vi "Required LV Version.vi"(8 "error in (no error)":errorcluster, 11 "Build Package Item in":refnum<class "Build Package Item.lvclass">) -> (0 "error out":errorcluster, 1 "64 Bit?":bool, 2 "LV Year":u32)   [LabVIEW 2019, in "VIPM.lvlib" / "Build Package Item.lvclass"]
uses:
  Build Package Item.lvclass
  <vilib>/xml/NI_XML.lvlib
  <vilib>/xml/Close Reference(Node).vi
  <vilib>/xml/Load XML File.vi
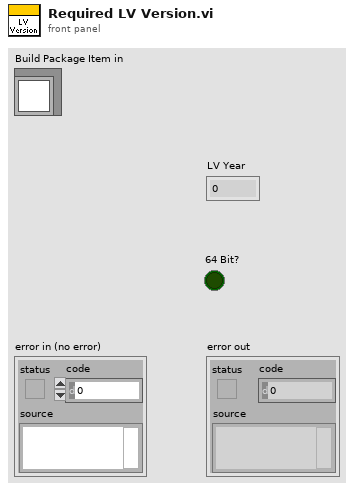
[diagram p1: front panel]
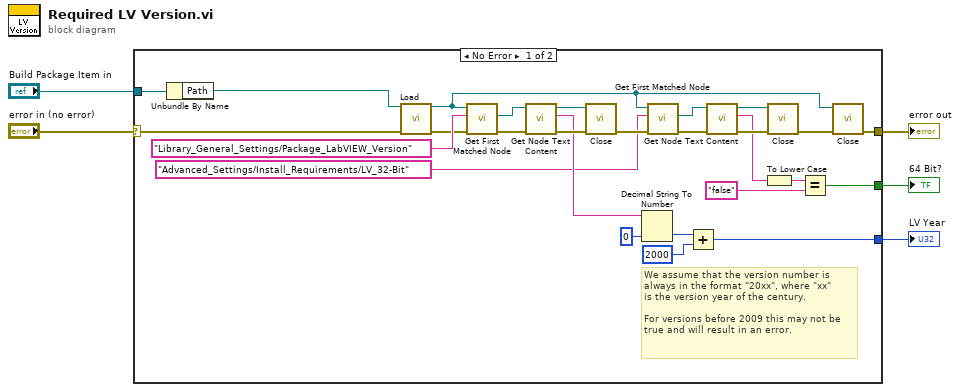
[diagram p0: block diagram]
diagram:
  n1 = case shown="No Error" "error in (no error)" {
    selector: "error in (no error)" -> [w25 w33]
    tunnel: [w24 w33] -> w4
    tunnel: [w20 _] -> w3
    tunnel: "Build Package Item in" -> [w19 _]
    tunnel: [w6 _] -> w1
    frame No Error {
      # "We assume that the version number is\nalways in the format \"20xx\", where \"xx\"\nis the version year of the century.\n\nFor versions before 2009 this may not be\ntrue and will result in an error."
      n2 = Unbundle By Name(w19) -> ("Path"=w18:path)
      n3 = call-poly <vilib>:"Load.vi"("path to XML document"=w18, "error in (no error)"=w25) -> ("DOM document out"=w10:refnum<k20>, "error out"=w31:errorcluster)  [unwired: 11 in, 1 out]
      n4 = call <vilib>:"Get First Matched Node.vi"("error in (no error)"=w31, "XPath expression"="Library_General_Settings/Package_LabVIEW_Version", "node in"=w10) -> ("error out"=w29:errorcluster, "node result"=w30:refnum<k20>)  [unwired: 6 in, 1 out]
      n5 = call <vilib>:"Get Node Text Content.vi"("error in (no error)"=w29, "node in"=w30) -> ("error out"=w28:errorcluster, "node text"=w26:string, "node out"=w27:refnum<k20>)  [unwired: 7 in]
      n6 = call-poly <vilib>:"Close.vi"("error in (no error)"=w28, "node"=w27) -> ("error out"=w16:errorcluster)  [unwired: 7 in]
      n7 = Decimal String To Number(string=w26, default (0L)=u32 0 ("default (0 I32)")) -> (number=w22:u32)  [unwired: 1 in, 1 out]
      n8 = call <vilib>:"Get First Matched Node.vi"("error in (no error)"=w16, "XPath expression"="Advanced_Settings/Install_Requirements/LV_32-Bit", "node in"=w10) -> ("error out"=w17:errorcluster, "node result"=w11:refnum<k20>)  [unwired: 6 in, 1 out]
      n9 = Add(x=w22, y=u32 2000) -> (x+y=w20:u32)
      n10 = call <vilib>:"Get Node Text Content.vi"("error in (no error)"=w17, "node in"=w11) -> ("error out"=w15:errorcluster, "node text"=w9:string, "node out"=w14:refnum<k20>)  [unwired: 7 in]
      n11 = To Lower Case(string=w9) -> (all lower case string=w8:string)
      n12 = call-poly <vilib>:"Close.vi"("error in (no error)"=w15, "node"=w14) -> ("error out"=w13:errorcluster)  [unwired: 7 in]
      n13 = Equal?(x=w8, y="false") -> (x = y?=w6:bool)
      n14 = call-poly <vilib>:"Close.vi"("error in (no error)"=w13, "node"=w10) -> ("error out"=w24:errorcluster)  [unwired: 7 in]
    }
    frame Error {
    }
  }
  "error out" <- w4
  "LV Year" <- w3
  "64 Bit?" <- w1
